vi "Keep position above object.vi"(7 "nr of particles":i32, 8 "bottom":dbl, 9 "right":dbl, 10 "top":dbl, 11 "left":dbl) -> (0 "Hover":bool, 1 "Roll":dbl format="%#_6f", 2 "Pitch":dbl format="%#_6f")   [LabVIEW 2014]
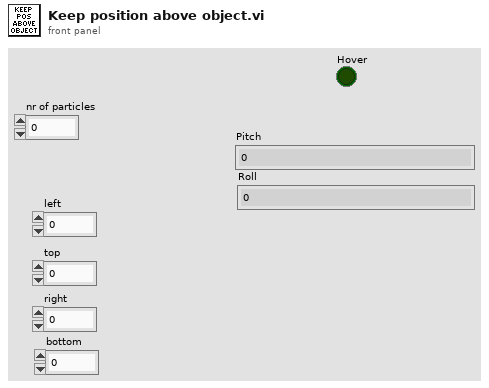
[diagram p1: front panel]
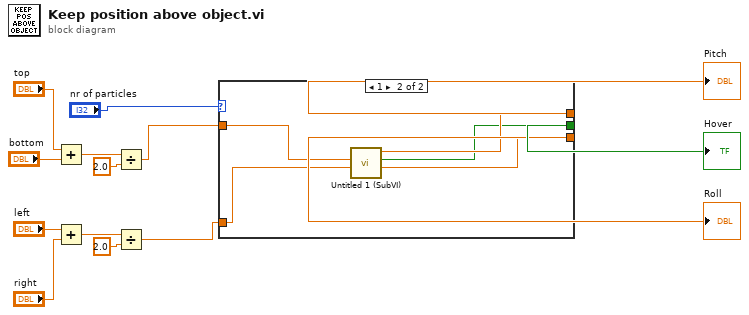
[diagram p0: block diagram]
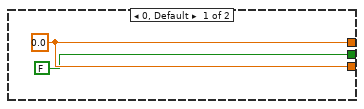
[diagram p2: hidden frame]
diagram:
  n1 = Add(x="top", y="bottom") -> (x+y=w8:dbl)
  n2 = Add(x="left", y="right") -> (x+y=w7:dbl)
  n3 = Divide(x=w8, y=2.0) -> (x/y=w6:dbl)
  n4 = Divide(x=w7, y=2.0) -> (x/y=w5:dbl)
  n5 = case shown="1" "nr of particles" {
    tunnel: w6 -> [_ w21]
    tunnel: w5 -> [_ w20]
    tunnel: [w16 w19] -> w4
    tunnel: [FALSE ("Hover") w18] -> w3
    tunnel: [w16 w17] -> w2
    frame 0, Default {
      w16 = 0.0 ("Pitch")
    }
    frame 1 {
      n6 = call "Untitled 1 (SubVI).vi"("X"=w20, "Y"=w21) -> ("Roll"=w17:dbl, "Hover"=w18:bool, "Pitch"=w19:dbl)  [unwired: 7 in]
    }
  }
  "Pitch" <- w4
  "Roll" <- w2
  "Hover" <- w3
